vi "Compile APU 1.3 Data.vi"(8 "error in (no error)":errorcluster, 11 "Device Item Ref in":T3 format="%.0x") -> (0 "error out":errorcluster, 2 "APUs":T1[](array[typedef]), 3 "Device Item Ref out":T3 format="%.0x")   [LabVIEW 2015, in "Engine Simulation Toolkit System Explorer.lvlib"]
uses:
  Engine Simulation Toolkit System Explorer.lvlib
  <vilib>/NI Veristand/Custom Device API/Custom Device Item Ref.ctl
  Shared/1.3 APU Engine Data.ctl
  Shared/1.0 APU Engine FIFO Idxs.ctl
  Shared/Properties.vi
  Shared/Constants and GUIDs.vi
  <vilib>/NI Veristand/Custom Device Tools/Custom Device Utility Library/NI VeriStand - Search for All Items by GUID.vi
  <vilib>/NI Veristand/Custom Device API/Get Item Property (String).vi
  <vilib>/NI Veristand/Custom Device API/Get Item Property (Double).vi
  <vilib>/NI Veristand/Custom Device API/Get Item Property (Boolean).vi
  <vilib>/NI Veristand/Custom Device API/Get Item Property (U16).vi
  <vilib>/NI Veristand/Custom Device Tools/Custom Device Utility Library/NI VeriStand - Search for Item by GUID.vi
  Shared/Engine Simulation Toolkit Shared.lvlib
  <vilib>/NI VeriStand/Custom Device API/Custom Device API.lvlib
  <vilib>/NI VeriStand/Custom Device Tools/Custom Device Utility Library/Custom Device Utility Library.lvlib
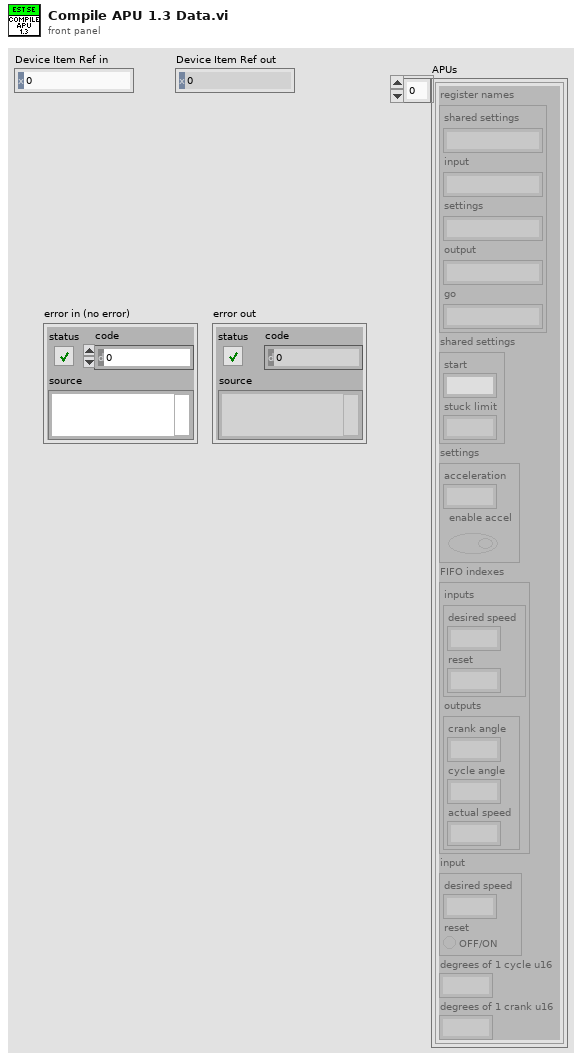
[diagram p1: front panel]
types:
  T1 = typedef "Engine Simulation Toolkit Shared.lvlib/1.3 APU Engine Data.ctl" = cluster{"register names":cluster{"shared settings":string, "input":string, "settings":string, "output":string, "go":string}, "shared settings":cluster{"start":fxp<+,17,17>, "stuck limit":fxp<+,18,18>}, "settings":cluster{"acceleration":fxp<+,18,-20>, "enable accel":bool}, "FIFO indexes":T2, "input":cluster{"desired speed":fxp<+/-,23,2>, "reset":bool}, "degrees of 1 cycle u16":dbl, "degrees of 1 crank u16":dbl}
  T2 = typedef "Engine Simulation Toolkit Shared.lvlib/1.0 APU Engine FIFO Idxs.ctl" = cluster{"inputs":cluster{"desired speed":i32, "reset":i32}, "outputs":cluster{"crank angle":i32, "cycle angle":i32, "actual speed":i32}}
  T3 = typedef "Custom Device API.lvlib/Custom Device Item Ref.ctl" = u64
  T4 = typedef "Engine Simulation Toolkit Shared.lvlib/Channel.ctl" = cluster{"Name":string, "Units":string, "Default":dbl, "Description":string, "Scalable":bool}
  T5 = cluster{"desired speed":fxp<+/-,23,2>, "reset":bool}
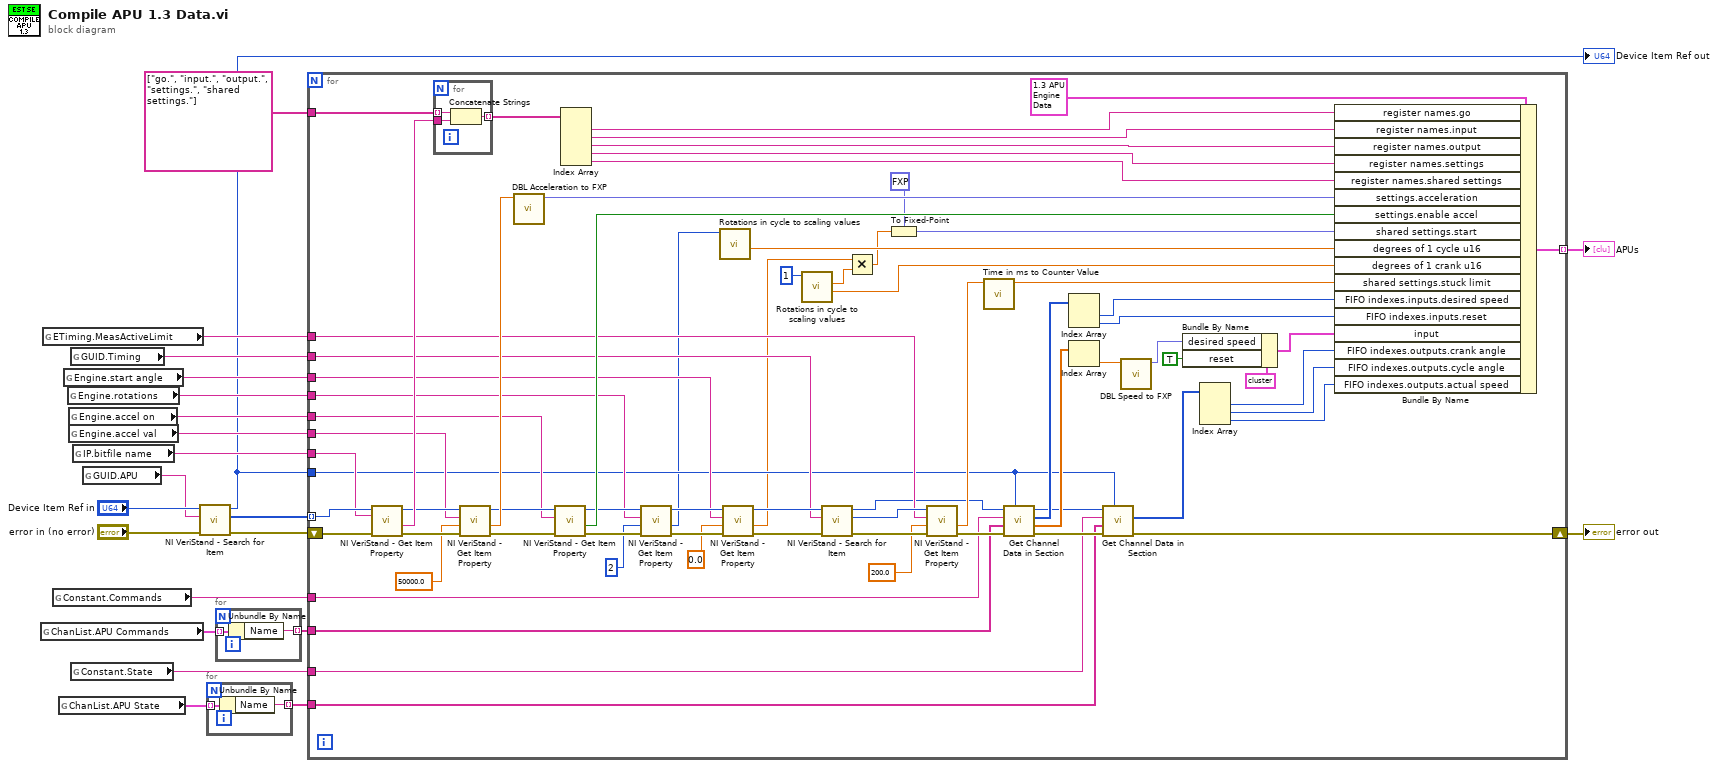
[diagram p0: block diagram]
diagram:
  n1 = global read "Constants and GUIDs.vi" "ChanList.APU Commands"() -> (w5:T4[])
  n2 = global read "Properties.vi" "ETiming.MeasActiveLimit"() -> (w10:string)
  n3 = global read "Constants and GUIDs.vi" "Constant.Commands"() -> (w9:string)
  n4 = global read "Constants and GUIDs.vi" "ChanList.APU State"() -> (w3:T4[])
  n5 = global read "Properties.vi" "Engine.start angle"() -> (w12:string)
  n6 = global read "Properties.vi" "Engine.rotations"() -> (w13:string)
  n7 = global read "Properties.vi" "Engine.accel on"() -> (w14:string)
  n8 = global read "Properties.vi" "Engine.accel val"() -> (w16:string)
  n9 = global read "Constants and GUIDs.vi" "GUID.Timing"() -> (w11:string)
  n10 = global read "Constants and GUIDs.vi" "Constant.State"() -> (w6:string)
  n11 = global read "Properties.vi" "IP.bitfile name"() -> (w18:string)
  n12 = global read "Constants and GUIDs.vi" "GUID.APU"() -> (w20:string)
  n13 = call-poly <vilib>:"NI VeriStand - Search for Item.vi"("error in"="error in (no error)", "Item GUID"=w20, "Section Ref in"="Device Item Ref in") -> ("error out"=w19:errorcluster, "Item Refs"=w1:T3[], "Section Ref out"=w7:T3)  [unwired: 5 in, 1 out]
  "Device Item Ref out" <- w7
  n14 = for {
    tunnel: w3 -> [w24] mode=indexing
    tunnel: [w23] -> w2 mode=indexing
    n15 = Unbundle By Name(w24) -> ("Name"=w23:string)
  }
  n16 = for {
    tunnel: w5 -> [w26] mode=indexing
    tunnel: [w25] -> w4 mode=indexing
    n17 = Unbundle By Name(w26) -> ("Name"=w25:string)
  }
  n18 = for {
    shift-right: [w51] -> w15
    shift-left: w19 -> [w98]
    tunnel: w1 -> [w97] mode=indexing
    tunnel: w18 -> [w96]
    tunnel: string[] ["go.", "input.", "output.", "settings.", "shared settings."] -> [w94]
    tunnel: w16 -> [w89]
    tunnel: w14 -> [w83]
    tunnel: w13 -> [w79]
    tunnel: w12 -> [w75]
    tunnel: w11 -> [w70]
    tunnel: w10 -> [w67]
    tunnel: w9 -> [w62]
    tunnel: w4 -> [w40]
    tunnel: [w56] -> w8 mode=indexing
    tunnel: w7 -> [w50]
    tunnel: w6 -> [w48]
    tunnel: w2 -> [w39]
    n19 = call-poly <vilib>:"NI VeriStand - Get Item Property.vi"("error in (no error)"=w98, "Property Name"=w96, "Item Ref in"=w97) -> ("error out"=w90:errorcluster, "Value"=w95:string, "Item Ref out"=w91:T3)  [unwired: 5 in, 1 out]
    n20 = for {
      tunnel: w95 -> [w101]
      tunnel: w94 -> [w100] mode=indexing
      tunnel: [w99] -> w92 mode=indexing
      n21 = Concatenate Strings(w100, w101) -> (w99:string)
    }
    n22 = call-poly <vilib>:"NI VeriStand - Get Item Property.vi"("error in (no error)"=w90, "Default Value"=50000.0, "Property Name"=w89, "Item Ref in"=w91) -> ("error out"=w88:errorcluster, "Value"=w87:dbl, "Item Ref out"=w84:T3)  [unwired: 4 in, 1 out]
    n23 = call "DBL Acceleration to FXP.vi"("Desired acceleration (RPM/sec)"=w87) -> ("FXP acceleration"=w86:fxp<+,18,-20>)  [unwired: 6 in, 4 out]
    n24 = call-poly <vilib>:"NI VeriStand - Get Item Property.vi"("error in (no error)"=w88, "Property Name"=w83, "Item Ref in"=w84) -> ("error out"=w85:errorcluster, "Value"=w82:bool, "Item Ref out"=w80:T3)  [unwired: 5 in, 1 out]
    n25 = Index Array(array=w92) -> (element #1=w38:string, element #2=w37:string, element #3=w36:string, element #4=w35:string, element #5=w34:string)  [unwired: 5 in]
    n26 = call-poly <vilib>:"NI VeriStand - Get Item Property.vi"("error in (no error)"=w85, "Default Value"=u16 2, "Property Name"=w79, "Item Ref in"=w80) -> ("error out"=w81:errorcluster, "Value"=w33:u16, "Item Ref out"=w76:T3)  [unwired: 4 in, 1 out]
    n27 = call "Rotations in cycle to scaling values.vi"("rotations in a cycle"=w33) -> ("degrees of one u16"=w32:dbl)  [unwired: 8 in, 2 out]
    n28 = call-poly <vilib>:"NI VeriStand - Get Item Property.vi"("error in (no error)"=w81, "Default Value"=0.0, "Property Name"=w75, "Item Ref in"=w76) -> ("error out"=w77:errorcluster, "Value"=w30:dbl, "Item Ref out"=w71:T3)  [unwired: 4 in, 1 out]
    n29 = call "Rotations in cycle to scaling values.vi"("rotations in a cycle"=u16 1) -> ("degrees of one u16"=w41:dbl, "angle to u16 scale factor"=w31:dbl)  [unwired: 8 in, 1 out]
    n30 = call-poly <vilib>:"NI VeriStand - Search for Item.vi"("error in"=w77, "Item GUID"=w70, "Section Ref in"=w71) -> ("error out"=w72:errorcluster, "Item Ref"=w68:T3, "Section Ref out"=w63:T3)  [unwired: 5 in, 1 out]
    n31 = Multiply(x=w30, y=w31) -> (x*y=w29:dbl)
    n32 = To Fixed-Point(fixed-point type=fxp<+,17,17> 0.0 ("shared settings.start"), number=w29) -> (fixed-point=w27:fxp<+,17,17>)
    n33 = call-poly <vilib>:"NI VeriStand - Get Item Property.vi"("error in (no error)"=w72, "Default Value"=200.0, "Property Name"=w67, "Item Ref in"=w68) -> ("error out"=w69:errorcluster, "Value"=w65:dbl)  [unwired: 4 in, 2 out]
    n34 = call "Time in ms to Counter Value.vi"("time (ms)"=w65) -> ("counter value"=w64:dbl)  [unwired: 10 in]
    n35 = call "Get Channel Data in Section.vi"("Custom device ref"=w50, "error in (no error)"=w69, "Channels"=w40, "Section (\"\":none)"=w62, "Item Ref in"=w63) -> ("error out"=w61:errorcluster, "default values"=w55:dbl[], "FIFO indexes"=w60:i32[], "Item Ref out"=w49:T3)  [unwired: 2 in, 1 out]
    n36 = Index Array(array=w60) -> (element #1=w59:i32, element #2=w58:i32)  [unwired: 2 in]
    n37 = Index Array(array=w55) -> (element=w54:dbl)  [unwired: 1 in]
    n38 = call "Get Channel Data in Section.vi"("Custom device ref"=w50, "error in (no error)"=w61, "Channels"=w39, "Section (\"\":none)"=w48, "Item Ref in"=w49) -> ("error out"=w51:errorcluster, "FIFO indexes"=w47:i32[])  [unwired: 2 in, 3 out]
    n39 = call "DBL Speed to FXP.vi"("Desired speed (RPM)"=w54) -> ("FXP speed"=w52:fxp<+/-,23,2>)  [unwired: 6 in, 4 out]
    n40 = Bundle By Name(cluster=T5 {"desired speed"=0.0, "reset"=FALSE} ("input"), "desired speed"=w52, "reset"=TRUE) -> (w53:T5)
    n41 = Index Array(array=w47) -> (element #1=w46:i32, element #2=w45:i32, element #3=w44:i32)  [unwired: 3 in]
    n42 = Bundle By Name(cluster=T1 {"register names"={"shared settings"="", "input"="", "settings"="", "output"="", "go"=""}, "shared settings"={"start"=0.0, "stuck limit"=0.0}, "settings"={"acceleration"=0.0, "enable accel"=FALSE}, "FIFO indexes"={"inputs"={"desired speed"=0, "reset"=0}, "outputs"={"crank angle"=0, "cycle angle"=0, "actual speed"=0}}, "input"={"desired speed"=0.0, "reset"=FALSE}, "degrees of 1 cycle u16"=0.0, "degrees of 1 crank u16"=0.0} ("1.0.0 APU"), "register names.go"=w38, "register names.input"=w37, "register names.output"=w36, "register names.settings"=w35, "register names.shared settings"=w34, "settings.acceleration"=w86, "settings.enable accel"=w82, "shared settings.start"=w27, "degrees of 1 cycle u16"=w32, "degrees of 1 crank u16"=w41, "shared settings.stuck limit"=w64, "FIFO indexes.inputs.desired speed"=w59, "FIFO indexes.inputs.reset"=w58, "input"=w53, "FIFO indexes.outputs.crank angle"=w46, "FIFO indexes.outputs.cycle angle"=w45, "FIFO indexes.outputs.actual speed"=w44) -> (w56:T1)
  }
  "error out" <- w15
  "APUs" <- w8
